vi "Peak_Detecting.vi"(7 "PNG output folder":path=path "C:/Users/ansom/Desktop/Agilent/PNG's From Graphs/B_BG_7to-7", 8 "Use File Offset":bool, 9 "length":i32, 10 "subset start index":i32, 11 "Folder or File":path=path "B:/SketchSET/SA03008H.20180718/116_SG_0.5to2inc0.1_0T_-450mVto50mIV_16.8BG_@2K") -> (2 "avg amplitude":dbl[](graph)=[0.00017536593406920355, 0.00020620122398447798, 0.00021284953333698925, 0.0002127393992579631, 0.00019813819263914397, 0.00018368555935057164, 0.00018682088150134314, 0.000193567197233025, 0.0002010727309038395, 0.00020975733899876757, 0.00022060276143130155, 0.0002300224955236294, 0.000239868522528151, 0.0002487635701803875, 0.00025766004947254335, 0.0002665991807521474], 3 "avg FWHM":dbl[](graph)=[57.0, 54.0, 54.0, 56.0, 58.0, 61.0, 61.0, 60.0, 60.0, 59.0, 59.0, 59.0, 58.0, 58.0, 58.0, 57.0])   [LabVIEW 2016]
uses:
  <vilib>/Analysis/baseanly.llb/Mean (DBL).vi
  <userlib>/LevyLab/LV to ITX/LVtoITX.lvclass
  <vilib>/Analysis/NI_AALBase.lvlib
panel:
  out "Waveform Graph":dbl[][](graph)=[[-0.010111200020844088, -0.013021275220844073, -0.011757919220843993, -0.01049456322084407, -0.009257345620844093, -0.007985276820844107, -0.006739346420844139, -0.005554405620844091, -0.0044043160208441234, -0.0036201640208441683, -0.0030625448208438217, -0.0025484896208490676, -0.0020692856208002334, -0.0016162200208775462, -0.0011892928247993555, -0.0007885039855493616], [-0.0, -0.0, -0.0, -0.0, -0.0, -0.0, -0.0, -0.0, -0.0, -0.0, -0.0, -0.0, -0.0, -0.0, -0.0, -0.0], [-0.0, -0.0, -0.0, -0.0, -0.0, -0.0, -0.0, -0.0, -0.0, -0.0, -0.0, -0.0, -0.0, -0.0, -0.0, -0.0]]
  out "x*y":dbl[][](array[numeric])=[[-0.010111200020844088, -0.0, -0.0], [-0.013021275220844073, -0.0, -0.0], [-0.011757919220843993, -0.0, -0.0], [-0.01049456322084407, -0.0, -0.0], [-0.009257345620844093, -0.0, -0.0], [-0.007985276820844107, -0.0, -0.0], [-0.006739346420844139, -0.0, -0.0], [-0.005554405620844091, -0.0, -0.0], [-0.0044043160208441234, -0.0, -0.0], [-0.0036201640208441683, -0.0, -0.0], [-0.0030625448208438217, -0.0, -0.0], [-0.0025484896208490676, -0.0, -0.0], [-0.0020692856208002334, -0.0, -0.0], [-0.0016162200208775462, -0.0, -0.0], [-0.0011892928247993555, -0.0, -0.0], [-0.0007885039855493616, -0.0, -0.0]]
  out "peak detection locations":dbl[][](array[numeric])=[[-0.2320998994776441], [-0.2988998994776438], [-0.2698998994776419], [-0.24089989947764373], [-0.21249989947764425], [-0.18329989947764455], [-0.1546998994776453], [-0.12749989947764417], [-0.10109989947764492], [-0.08309989947764596], [-0.070299899477638], [-0.05849989947775842], [-0.047499899476637436], [-0.037099899478412135], [-0.027299899568436224], [-0.01809989866746308]]
  out "size(s)":i32=2399
  out "final FWHM mean for this folder":dbl=58.0625 format="%p"
  out "final amplitude mean for this folder":dbl=0.00021523216069771782 format="%p"
  out "Chopped IV":cluster{dbl[], dbl[]}(graph)
  out "Chopped dI/dV":T1(graph)
  out "input data":cluster{dbl[], dbl[]}[](graph)
  in  "Peak Threshold":dbl=1e-08 format="%p"
  in  "Diff bin size":dbl=2.0
  in  "Points to chop off the bottom edge":i32=50
  in  "Points to chop off the top edge":i32=50
  out "Iterations of loop":i32=15
  out "directory":bool=TRUE
  out "Comments":string="IGOR\nX// Date: 7/20/2018 2:10 PM\nX// SA03008H\nX// 2K\nX// Source 2 Drain 28 (lockin 2 and 7)\nX// \nX// constant \nX// \nX// Sweeping SG 0.5 to 1.5 inc 01\nX// \nX// Gohm resistor in SG1 now (KH1), sweep SG\nX// \nX// 250mV AC -200mV DC for the IV sweep\nX// \nX// 0T\n\nX// DSA_Vsg1=2.000000\n\nX// \nX// B= 0.000001\n\n\n\n\n\n\n\n\n\n\n\n\n\n\n\n\n\n\n\n\n\n\n\n\n\n\n\n\n\n\n\n\n\n\n\n\n\n\n\n\nX \nX Display/R 'time.SA03008H.20180718.000015'\nX AppendToGraph 'temp.SA03008H.20180718.000015'\nX AppendToGraph 'B.SA03008H.20180718.000015'\nX AppendToGraph 'Vsource.SA03008H.20180718.000015'\nX AppendToGraph 'Lockin0.SA03008H.20180718.000015'\nX AppendToGraph 'Lockin1.SA03008H.20180718.000015'\nX AppendToGraph 'Lockin2.SA03008H.20180718.000015'\nX AppendToGraph 'Lockin3.SA03008H.20180718.000015'\nX AppendToGraph 'Lockin4.SA03008H.20180718.000015'\nX AppendToGraph 'Lockin5.SA03008H.20180718.000015'\nX AppendToGraph 'B_rate.SA03008H.20180718.000015'\nX AppendToGraph 'DC0.SA03008H.20180718.000015'\nX AppendToGraph 'DC1.SA03008H.20180718.000015'\nX AppendToGraph 'DC2.SA03008H.20180718.000015'\nX AppendToGraph 'DC3.SA03008H.20180718.000015'\nX AppendToGraph 'DC4.SA03008H.20180718.000015'\nX AppendToGraph 'DC5.SA03008H.20180718.000015'\nX AppendToGraph 'DC6.SA03008H.20180718.000015'\nX AppendToGraph 'DC7.SA03008H.20180718.000015'\nX Label bottom \"x label\"\nX Label left \"y label\"\nX ModifyGraph rgb('time.SA03008H.20180718.000015')=(65280,0,0)\nX ModifyGraph rgb('temp.SA03008H.20180718.000015')=(65280,18432,0)\nX ModifyGraph rgb('B.SA03008H.20180718.000015')=(65280,36864,0)\nX ModifyGraph rgb('Vsource.SA03008H.20180718.000015')=(65280,55296,0)\nX ModifyGraph rgb('Lockin0.SA03008H.20180718.000015')=(57344,65280,0)\nX ModifyGraph rgb('Lockin1.SA03008H.20180718.000015')=(37376,65280,0)\nX ModifyGraph rgb('Lockin2.SA03008H.20180718.000015')=(18944,65280,0)\nX ModifyGraph rgb('Lockin3.SA03008H.20180718.000015')=(512,65280,0)\nX ModifyGraph rgb('Lockin4.SA03008H.20180718.000015')=(0,65280,17920)\nX ModifyGraph rgb('Lockin5.SA03008H.20180718.000015')=(0,65280,36352)\nX ModifyGraph rgb('B_rate.SA03008H.20180718.000015')=(0,65280,54784)\nX ModifyGraph rgb('DC0.SA03008H.20180718.000015')=(0,57856,65280)\nX ModifyGraph rgb('DC1.SA03008H.20180718.000015')=(0,39424,65280)\nX ModifyGraph rgb('DC2.SA03008H.20180718.000015')=(0,20992,65280)\nX ModifyGraph rgb('DC3.SA03008H.20180718.000015')=(0,2560,65280)\nX ModifyGraph rgb('DC4.SA03008H.20180718.000015')=(17408,0,65280)\nX ModifyGraph rgb('DC5.SA03008H.20180718.000015')=(35840,0,65280)\nX ModifyGraph rgb('DC6.SA03008H.20180718.000015')=(54272,0,65280)\nX ModifyGraph rgb('DC7.SA03008H.20180718.000015')=(65280,0,58368)\nX Legend/C/N=text0/J \"\\\\s('time.SA03008H.20180718.000015') time\\r\\\\s('temp.SA03008H.20180718.000015') temp\\r\\\\s('B.SA03008H.20180718.000015') B\\r\\\\s('Vsource.SA03008H.20180718.000015') Vsource\\r\\\\s('Lockin0.SA03008H.20180718.000015') Lockin0\\r\\\\s('Lockin1.SA03008H.20180718.000015') Lockin1\\r\\\\s('Lockin2.SA03008H.20180718.000015') Lockin2\\r\\\\s('Lockin3.SA03008H.20180718.000015') Lockin3\\r\\\\s('Lockin4.SA03008H.20180718.000015') Lockin4\\r\\\\s('Lockin5.SA03008H.20180718.000015') Lockin5\\r\\\\s('B_rate.SA03008H.20180718.000015') B_rate\\r\\\\s('DC0.SA03008H.20180718.000015') DC0\\r\\\\s('DC1.SA03008H.20180718.000015') DC1\\r\\\\s('DC2.SA03008H.20180718.000015') DC2\\r\\\\s('DC3.SA03008H.20180718.000015') DC3\\r\\\\s('DC4.SA03008H.20180718.000015') DC4\\r\\\\s('DC5.SA03008H.20180718.000015') DC5\\r\\\\s('DC6.SA03008H.20180718.000015') DC6\\r\\\\s('DC7.SA03008H.20180718.000015') DC7\"\nX ModifyGraph mirror(bottom)=1\nX ModifyGraph width=216\nX ModifyGraph height={Aspect,0.6}\nX ModifyGraph Log(bottom)=0\nX ModifyGraph Log(left)=0\nX \n"
  out "N__":cluster{"N1":dbl, "N2":dbl, "N3":dbl, "N4":dbl}={"N1"=3614955043.131174, "N2"=3614955043.131174, "N3"=3614955043.131174, "N4"=3614955043.131174} {"N4" format="%#_6p"; "N3" format="%#_6p"; "N2" format="%#_6p"; "N1" format="%#_6p"}
  in  "index":T2={"A"=5, "B"=3, "C"=2, "D"=0, "E"=3, "N1"=0, "N2"=0, "N3"=0, "N4"=0}
  # "50 ,  50"
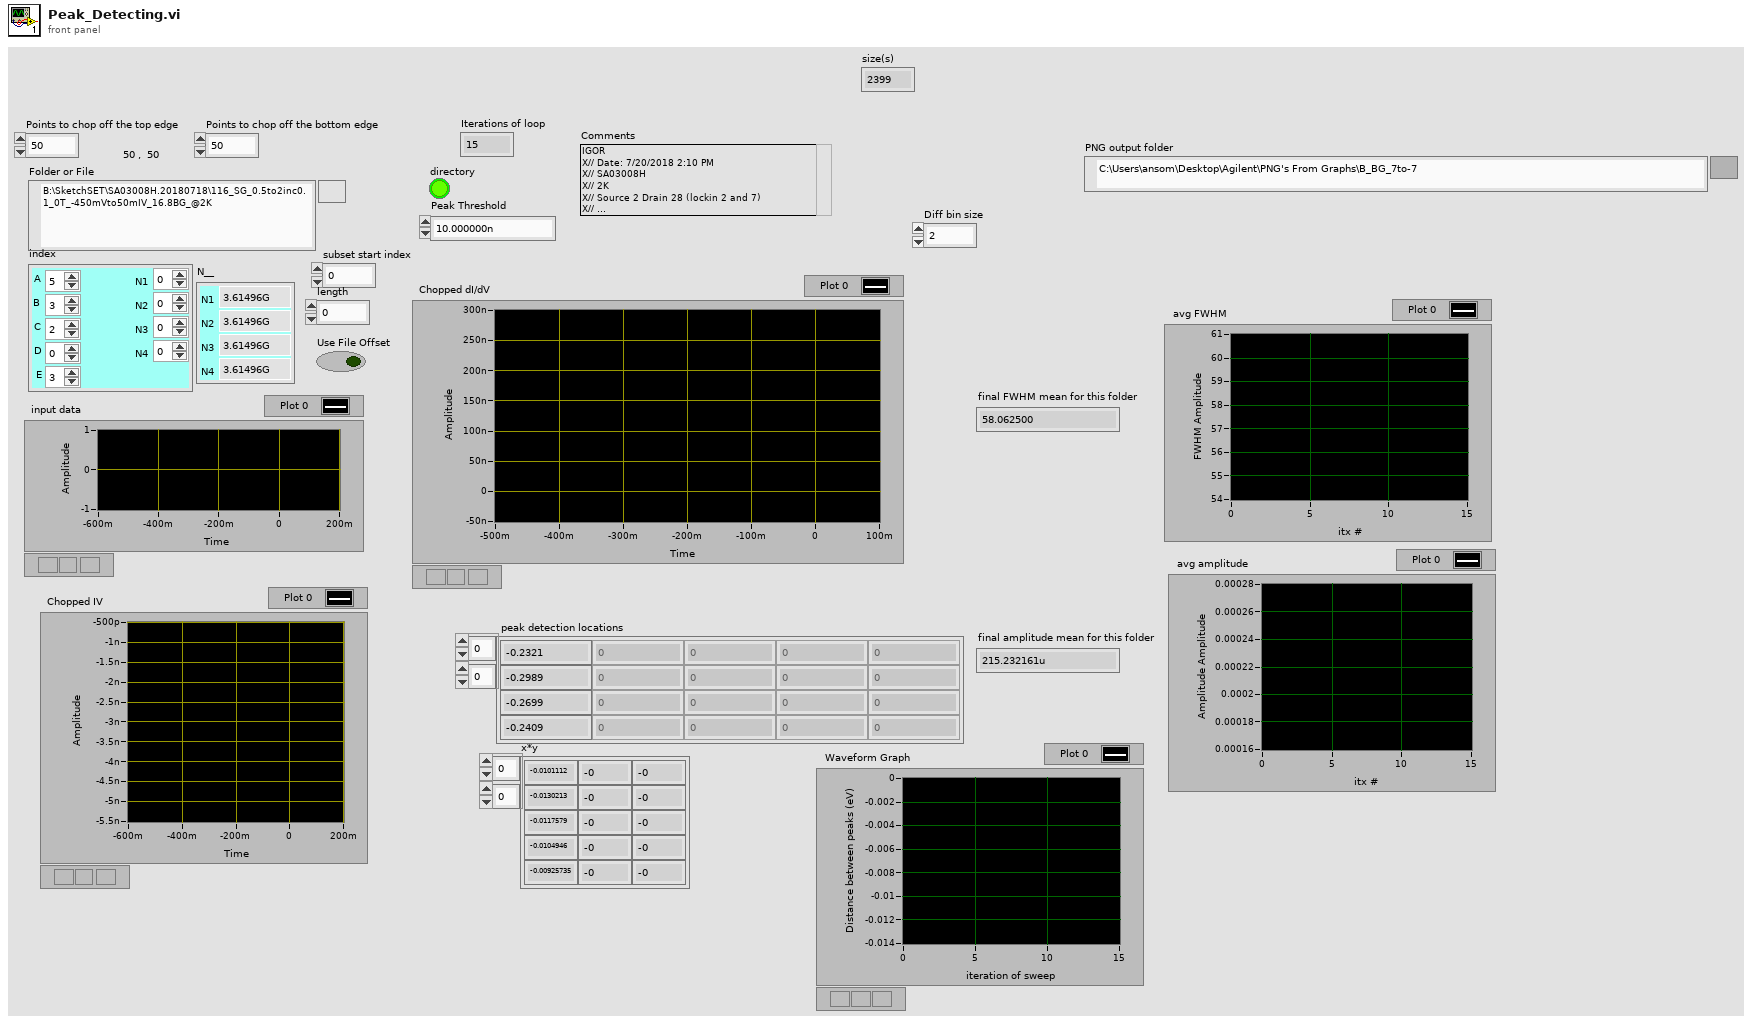
[diagram p1: front panel]
types:
  T1 = cluster{"Vsrc values":dbl[], "dI/dV values":dbl[]}
  T2 = cluster{"A":i32, "B":i32, "C":i32, "D":i32, "E":i32, "N1":i32, "N2":i32, "N3":i32, "N4":i32}
  T3 = cluster{"Decimated Array":dbl[], "Decimated Array":dbl[]}[]
  T4 = typedef "imagedata.ctl" = cluster{"image type":i32, "image depth":i32, "image":u8[], "mask":u8[], "colors":u32[], "Rectangle":cluster{"left":i16, "top":i16, "right":i16, "bottom":i16}}
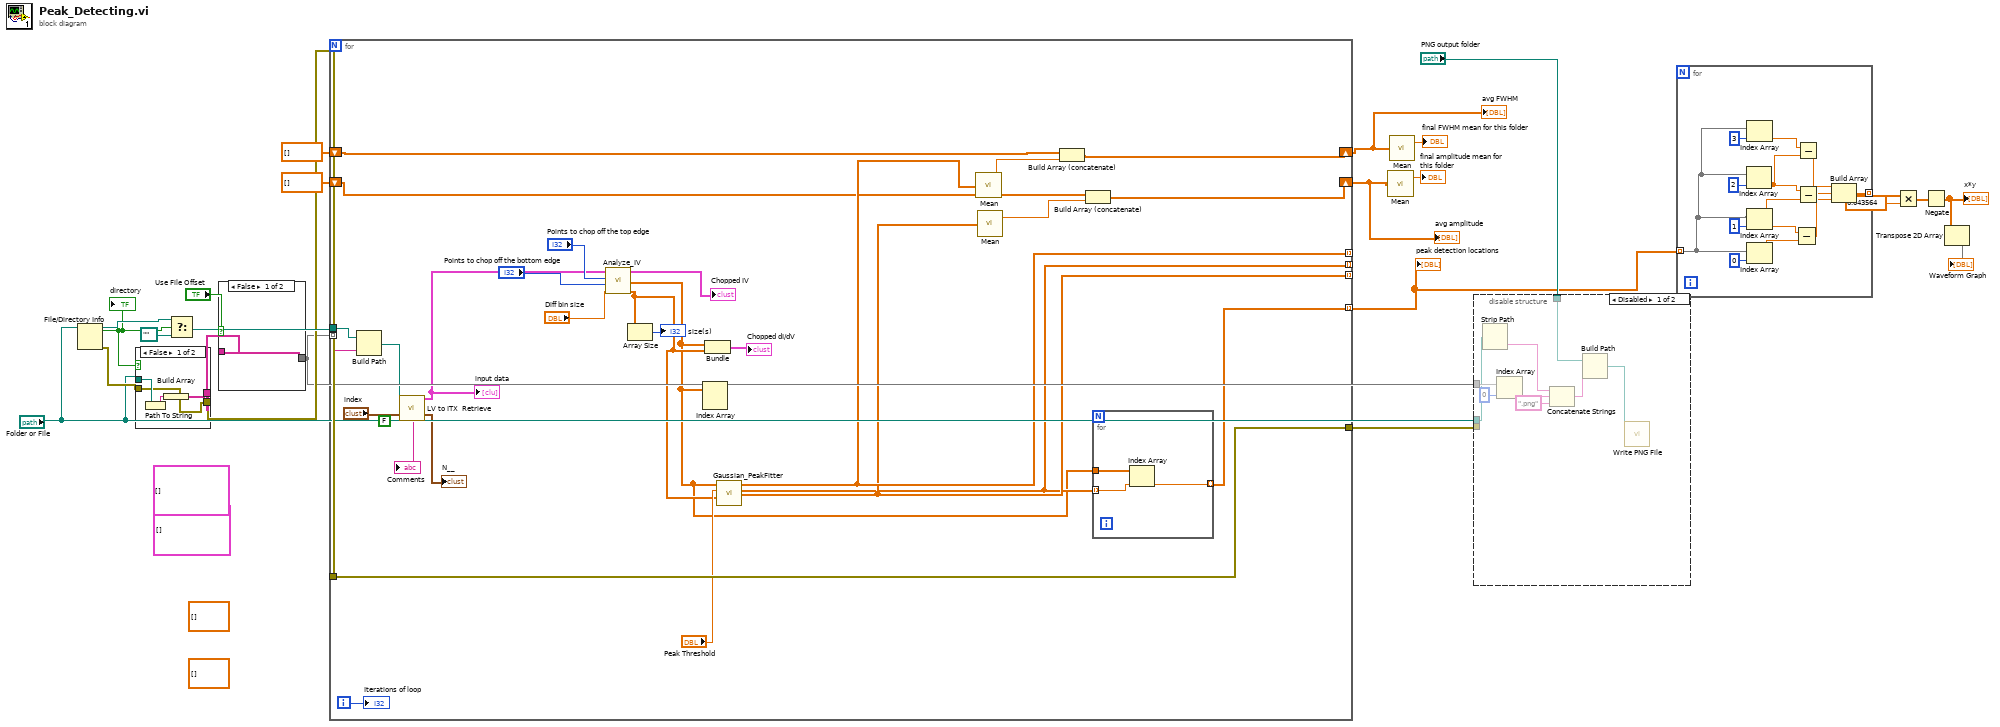
[diagram p0: block diagram]
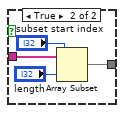
[diagram p3: hidden frame]
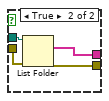
[diagram p4: hidden frame]
diagram:
  (unwired) dbl[][] []
  (unwired) dbl[][] []
  (unwired) T3 []
  (unwired) cluster{dbl[], dbl[]}[] []
  n1 = File/Directory Info(path="Folder or File") -> (path out=w23:path, directory=w22:bool, error out=w24:errorcluster)  [unwired: 1 in, 4 out]
  "directory" <- w22
  n2 = case shown="False" w22 {
    tunnel: "Folder or File" -> [w28 w32]
    tunnel: w24 -> [w25 w31]
    tunnel: [w26 w30] -> w19
    tunnel: [w25 w29] -> w18
    frame False {
      n3 = Path To String(path=w28) -> (string=w27:string)
      n4 = Build Array(w27) -> (w26:string[])
    }
    frame True {
      n5 = List Folder(path=w32, error in=w31) -> (filenames=w30:string[], error out=w29:errorcluster)  [unwired: 2 in, 2 out]
    }
  }
  n6 = Select(t=w23, s=w22, f=path "") -> (s? t:f=w21:path)
  n7 = case shown="False" "Use File Offset" {
    tunnel: w19 -> [w33 w37]
    tunnel: [w33 w36] -> w17
    frame False {
    }
    frame True {
      n8 = Array Subset(array=w37, index="subset start index", length="length") -> (w36:string[])
    }
  }
  n9 = for {
    tunnel: w17 -> [w62] mode=indexing
    tunnel: w21 -> [w60]
    tunnel: [w58] -> w15
    tunnel: w18 -> [w58]
    shift-right: [w48] -> w8
    shift-left: dbl[] [] -> [w46]
    shift-right: [w43] -> w9
    shift-left: dbl[] [] -> [w45]
    tunnel: [w50] -> _ mode=indexing
    tunnel: [w49] -> _ mode=indexing
    tunnel: [w41] -> _ mode=indexing
    tunnel: [w39] -> w6 mode=indexing
    i -> [w59]
    (unwired) FALSE ("stop")
    n10 = Build Path(base path=w60, name or relative path=w62) -> (appended path=w61:path)
    n11 = call <userlib>:"LV to ITX  Retrieve.vi"("File or Folder Path"=w61, "index"="index") -> ("A vs B"=w53:cluster{dbl[], dbl[]}[], "N"=→"N__":cluster{"N1":dbl, "N2":dbl, "N3":dbl, "N4":dbl}, "Comments"=→"Comments":string)  [unwired: 9 in, 2 out]
    "input data" <- w53
    n12 = call "Analyze_IV.vi"("Diff bin size"="Diff bin size", "Points to chop off the bottom edge"="Points to chop off the bottom edge", "Points to chop off the top edge"="Points to chop off the top edge", "A vs B IN"=w53) -> ("dI/dV values"=w40:dbl[], "Vsrc values"=w38:dbl[], "IV curve subsection"=→"Chopped IV":cluster{dbl[], dbl[]})  [unwired: 4 in, 1 out]
    n13 = Array Size(array=w40) -> (size(s)=→"size(s)":i32)
    n14 = Index Array(array=w38) -> ()  [unwired: 2 in, 2 out]
    n15 = Bundle("Vsrc values"=w38, "dI/dV values"=w40) -> (→"Chopped dI/dV":T1)  [unwired: 1 in]
    n16 = call "Gaussian_PeakFitter.vi"("Y array in"=w40, "Peak Threshold"="Peak Threshold", "X array in"=w38) -> ("Amplitudes"=w49:dbl[], "peak detection locations"=w41:dbl[], "FWHM, indices?"=w50:dbl[])  [unwired: 6 in]
    n17 = call-poly <vilib>:"Mean.vi"("X"=w50) -> ("mean"=w47:dbl)  [unwired: 1 out]
    n18 = call-poly <vilib>:"Mean.vi"("X"=w49) -> ("mean"=w44:dbl)  [unwired: 1 out]
    n19 = Build Array (concatenate)(w46, w47) -> (w48:dbl[])
    n20 = Build Array (concatenate)(w45, w44) -> (w43:dbl[])
    n21 = for {
      tunnel: w41 -> [w68] mode=indexing
      tunnel: w38 -> [w67]
      tunnel: [w66] -> w39 mode=indexing
      n22 = Index Array(array=w67, index=w68) -> (element=w66:dbl)
    }
    "Iterations of loop" <- w59
  }
  "avg amplitude" <- w9
  "avg FWHM" <- w8
  "peak detection locations" <- w6
  n23 = call-poly <vilib>:"Mean.vi"("X"=w9) -> ("mean"=→"final amplitude mean for this folder":dbl)  [unwired: 1 out]
  n24 = call-poly <vilib>:"Mean.vi"("X"=w8) -> ("mean"=→"final FWHM mean for this folder":dbl)  [unwired: 1 out]
  n25 = disable-structure shown="Disabled" {
    disable-tunnel: w17 -> [w80 _]
    disable-tunnel: "PNG output folder" -> [w78 _]
    disable-tunnel: w15 -> [w76 _]
    disable-tunnel: "Folder or File" -> [w69 _]
    frame Disabled {
      n26 = Strip Path(path=w69) -> (name=w70:string)  [unwired: 1 out]
      n27 = Index Array(array=w80, index=0) -> (element=w73:string)
      n28 = Concatenate Strings(w70, w73, ".png" ("string")) -> (w72:string)
      n29 = Build Path(base path=w78, name or relative path=w72) -> (appended path=w79:path)
      n30 = call <vilib>:"Write PNG File.vi"("path to PNG file"=w79) -> ("error in (no error)"=w74:errorcluster, "image data"=w75:T4)  [unwired: 7 in, 2 out]
    }
    frame Enabled {
    }
  }
  n31 = for {
    tunnel: w6 -> [w92] mode=indexing
    tunnel: [w84] -> w4 mode=indexing
    n32 = Index Array(array=w92, index=2) -> (element=w86:dbl)
    n33 = Index Array(array=w92, index=3) -> (element=w87:dbl)
    n34 = Index Array(array=w92, index=1) -> (element=w85:dbl)
    n35 = Index Array(array=w92, index=0) -> (element=w93:dbl)
    n36 = Subtract(x=w85, y=w93) -> (x-y=w83:dbl)
    n37 = Subtract(x=w87, y=w86) -> (x-y=w82:dbl)
    n38 = Subtract(x=w86, y=w85) -> (x-y=w81:dbl)
    n39 = Build Array(w83, w81, w82) -> (w84:dbl[])
  }
  n40 = Multiply(x=w4, y=0.043564) -> (x*y=w3:dbl[][])
  n41 = Negate(x=w3) -> (-x=w2:dbl[][])
  "x*y" <- w2
  n42 = Transpose 2D Array(2D array=w2) -> (transposed array=→"Waveform Graph":dbl[][])
